vi "cDAQ v to value converter.vi"(7 "offset":dbl[](array[numeric]), 8 "error in (no error)":errorcluster, 9 "Max Value of cDAQ":dbl[](array[numeric]), 10 "Max Range":dbl[](array[numeric]), 11 "Voltage Input":dbl[](array[numeric])) -> (0 "error out":errorcluster, 3 "output value":dbl[](array[numeric]))   [LabVIEW 2019]
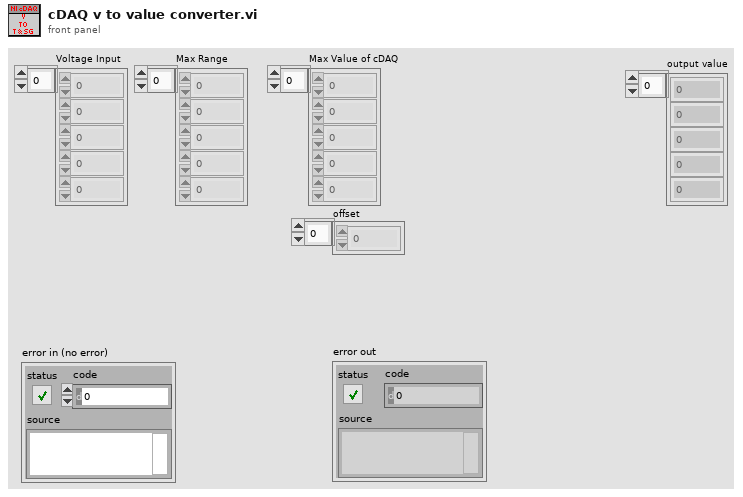
[diagram p1: front panel]
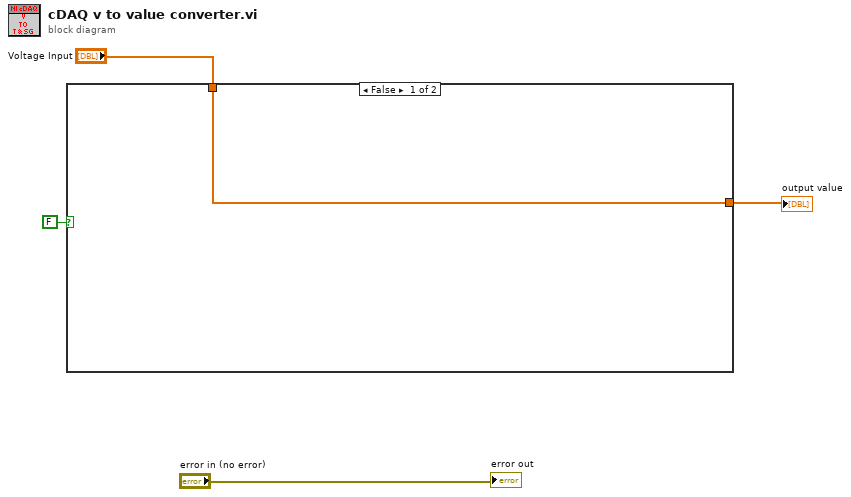
[diagram p0: block diagram]
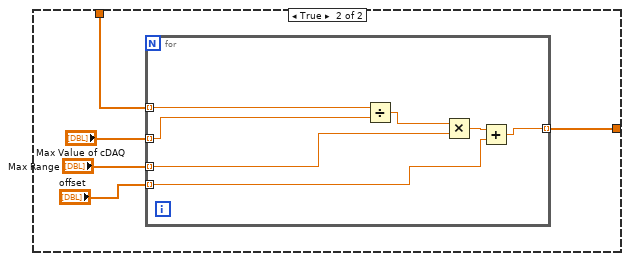
[diagram p2: hidden frame]
diagram:
  n1 = case shown="False" FALSE {
    tunnel: "Voltage Input" -> [w5 w10]
    tunnel: [w5 w9] -> w2
    frame False {
    }
    frame True {
      n2 = for {
        tunnel: w10 -> [w16] mode=indexing
        tunnel: [w14] -> w9 mode=indexing
        tunnel: "Max Value of cDAQ" -> [w13] mode=indexing
        tunnel: "Max Range" -> [w12] mode=indexing
        tunnel: "offset" -> [w11] mode=indexing
        n3 = Divide(x=w16, y=w13) -> (x/y=w17:dbl)
        n4 = Multiply(x=w17, y=w12) -> (x*y=w15:dbl)
        n5 = Add(x=w15, y=w11) -> (x+y=w14:dbl)
      }
    }
  }
  "output value" <- w2
  "error out" <- "error in (no error)"
